vi "Measurement.TestLauncher.vi"() -> ()   [LabVIEW 2017]
doc: "JKI State Machine Objects (SMO) 1.0.0.5\nJKI - JKI\nCopyright (c) 2016, JKI"
uses:
  Measurement.Free.UI.lvclass
  D:/Program Files (x86)/National Instruments/LabVIEW 2017/vi.lib/JKI/JKI SMO/SMO/SMO.lvclass
  D:/Program Files (x86)/National Instruments/LabVIEW 2017/vi.lib/JKI/JKI SMO/SMO.UI/SMO.UI.lvclass
  Measurement.Free/Measurement.Free.lvclass
  Measurement.Free/Typedefs/Configuration--Cluster.ctl
  <vilib>/JKI/JKI SMO/SMO/SMO.lvclass
  <vilib>/JKI/JKI SMO/SMO.UI/SMO.UI.lvclass
panel:
  in  "Stop":bool
  # "SMO UI Test Launcher"
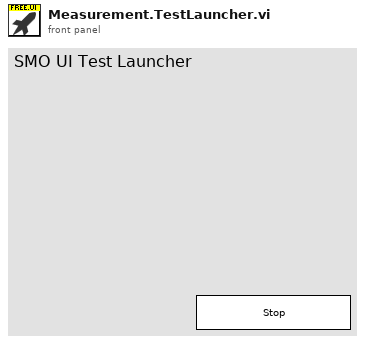
[diagram p1: front panel]
types:
  T1 = typedef "Measurement.Free.lvclass/Configuration--Cluster.ctl" = cluster{"Suffix":string}
  T2 = cluster{"SMO out":refnum<class "Measurement.Free.lvclass">}
  T3 = typedef "SMO.lvclass/Public Events.ctl" = cluster{"Error":refnum<user-event>, "State":refnum<user-event>, "Reserve State":refnum<user-event>}
  T4 = cluster{"Measurement.Free Public Events":refnum<event-registration>, "SMO.UI Public Events":refnum<event-registration>, "Event Registration Refnum":refnum<event-registration>}
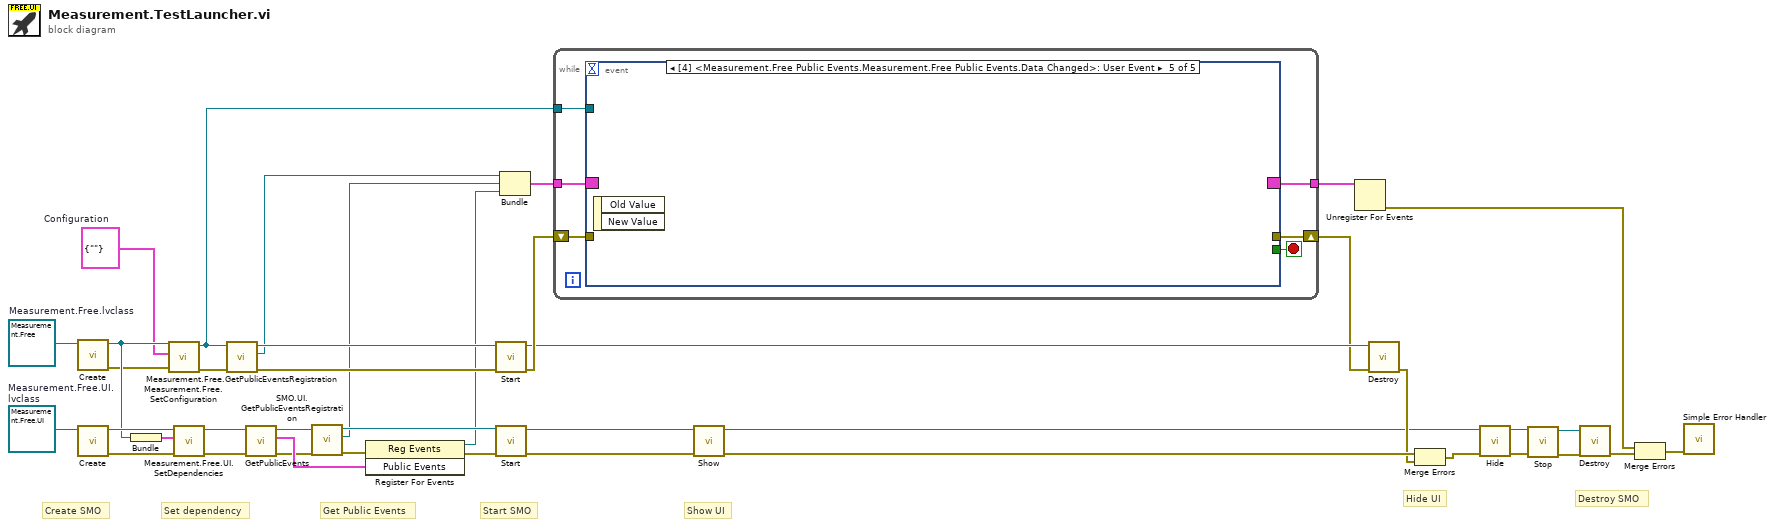
[diagram p0: block diagram]
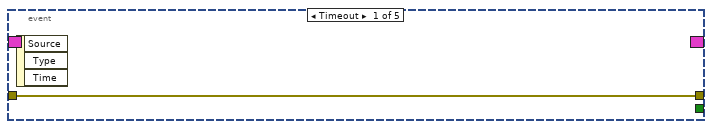
[diagram p2: hidden frame]
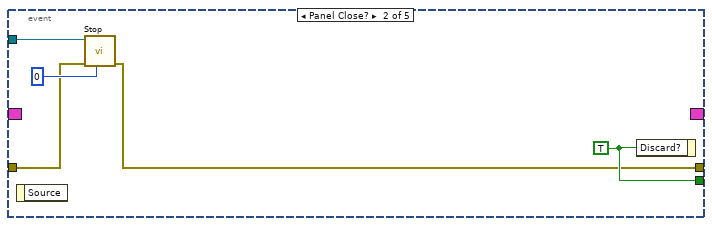
[diagram p3: hidden frame]
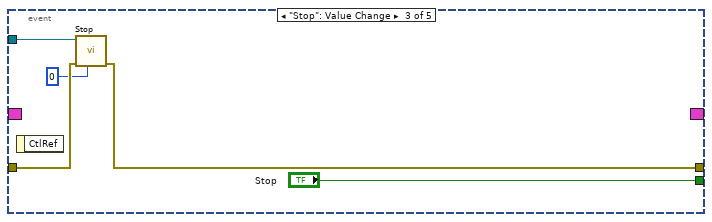
[diagram p4: hidden frame]
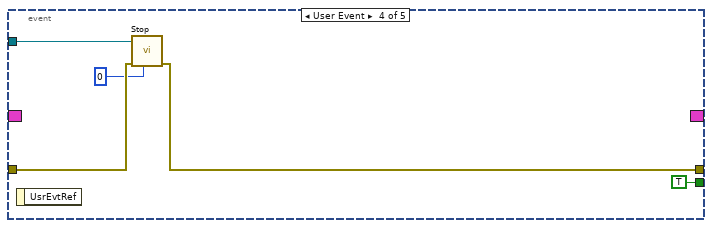
[diagram p5: hidden frame]
diagram:
  w25 = T1 {"Suffix"=""}  # Configuration
  w33 = refnum<class "Measurement.Free.lvclass"> refnum  # Measurement.Free.lvclass
  w34 = refnum<class "Measurement.Free.UI.lvclass"> refnum  # Measurement.Free.UI.lvclass
  # "Set dependency"
  # "Hide UI"
  # "Show UI"
  # "Get Public Events"
  # "Start SMO"
  # "Destroy SMO"
  # "Create SMO"
  n1 = call <vilib>:"Create.vi"("SMO"=w33) -> ("error out"=w26:errorcluster, "SMO out"=w27:refnum<class "Measurement.Free.lvclass">)  [unwired: 8 in, 1 out]
  n2 = call <vilib>:"Create.vi"("SMO"=w34) -> ("error out"=w30:errorcluster, "SMO out"=w32:refnum<class "Measurement.Free.UI.lvclass">)  [unwired: 8 in, 1 out]
  n3 = Bundle("SMO out"=w27) -> (w31:T2)  [unwired: 1 in]
  n4 = call "Measurement.Free.SetConfiguration.vi"("error in (no error)"=w26, "Configuration"=w25, "Measurement.Free"=w27) -> ("error out"=w10:errorcluster, "Measurement.Free out"=w11:refnum<class "Measurement.Free.lvclass">)  [unwired: 7 in]
  n5 = call "Measurement.Free.UI.SetDependencies.vi"("error in (no error)"=w30, "Dependencies"=w31, "Measurement.Free.UI in"=w32) -> ("error out"=w28:errorcluster, "Measurement.Free.UI out"=w29:refnum<class "Measurement.Free.UI.lvclass">)  [unwired: 7 in]
  n6 = call "Measurement.Free.GetPublicEventsRegistration.vi"("error in (no error)"=w10, "Measurement.Free"=w11) -> ("error out"=w8:errorcluster, "Measurement.Free Public Events"=w7:refnum<event-registration>, "Measurement.Free out"=w9:refnum<class "Measurement.Free.lvclass">)  [unwired: 7 in]
  n7 = call <vilib>:"GetPublicEvents.vi"("error in (no error)"=w28, "SMO"=w29) -> ("error out"=w5:errorcluster, "Public Events"=w35:T3, "SMO out"=w6:refnum<class "Measurement.Free.UI.lvclass">)  [unwired: 7 in]
  n8 = call <vilib>:"SMO.UI.GetPublicEventsRegistration.vi"("error in (no error)"=w5, "SMO.UI"=w6) -> ("error out"=w3:errorcluster, "SMO.UI Public Events"=w1:refnum<event-registration>, "SMO.UI out"=w4:refnum<class "Measurement.Free.UI.lvclass">)  [unwired: 7 in]
  n9 = register-events(error in=w3, w35) -> (reference out=w2:refnum<event-registration>, error out=w36:errorcluster)  [unwired: 1 in]
  n10 = call <vilib>:"Start.vi"("error in (no error)"=w8, "SMO"=w9) -> ("error out"=w22:errorcluster, "SMO out"=w21:refnum<class "Measurement.Free.lvclass">)  [unwired: 8 in]
  n11 = call <vilib>:"Start.vi"("error in (no error)"=w36, "SMO"=w4) -> ("error out"=w38:errorcluster, "SMO out"=w39:refnum<class "Measurement.Free.UI.lvclass">)  [unwired: 8 in]
  n12 = Bundle("Measurement.Free Public Events"=w7, "SMO.UI Public Events"=w1, "Event Registration Refnum"=w2) -> (w24:T4)  [unwired: 1 in]
  n13 = while {
    shift-right: [w46] -> w20
    shift-left: w22 -> [w45]
    tunnel: w24 -> [w42]
    tunnel: [w44] -> w23
    tunnel: w11 -> [w43]
    stop <- w47 stop-if-true
    n14 = event shown="[4] <Measurement.Free Public Events.Measurement.Free Public Events.Data Changed>: User Event" {
      selector: w42 -> [_ _ _ _ _]
      dyn-events: [_ _ _ _ _] -> w44
      timeout: _ -> [_ _ _ _ _]
      tunnel: [_ w53 "Stop" TRUE ("OK") _] -> w47
      tunnel: w43 -> [_ w52 w57 w63 _]
      tunnel: [w48 w49 w55 w61 _] -> w46
      tunnel: w45 -> [w48 w50 w56 w62 _]
      event Timeout {
        n15 = event-data() -> ()  [unwired: 1 in, 3 out]
      }
      event Panel Close? {
        w53 = TRUE ("OK")
        n16 = event-data() -> ()  [unwired: 1 in, 1 out]
        n17 = call <vilib>:"Stop.vi"("timeout in ms (-1)"=0, "error in (no error)"=w50, "SMO"=w52) -> ("error out"=w49:errorcluster)  [unwired: 7 in, 1 out]
        n18 = event-data("Discard?"=w53) -> ()  [unwired: 1 in, 1 out]
      }
      event "Stop": Value Change {
        n19 = event-data() -> ()  [unwired: 1 in, 1 out]
        n20 = call <vilib>:"Stop.vi"("timeout in ms (-1)"=0, "error in (no error)"=w56, "SMO"=w57) -> ("error out"=w55:errorcluster)  [unwired: 7 in, 1 out]
      }
      event User Event {
        n21 = event-data() -> ()  [unwired: 1 in, 1 out]
        n22 = call <vilib>:"Stop.vi"("timeout in ms (-1)"=0, "error in (no error)"=w62, "SMO"=w63) -> ("error out"=w61:errorcluster)  [unwired: 7 in, 1 out]
      }
      event User Event {
        n23 = event-data() -> ()  [unwired: 1 in, 2 out]
      }
    }
  }
  n24 = call <vilib>:"Show.vi"("error in (no error)"=w38, "SMO.UI"=w39) -> ("error out"=w37:errorcluster, "SMO.UI out"=w18:refnum<class "Measurement.Free.UI.lvclass">)  [unwired: 8 in]
  n25 = Unregister For Events(event registration refnum=w23) -> (error out=w41:errorcluster)  [unwired: 1 in]
  n26 = call <vilib>:"Destroy.vi"("error in (no error)"=w20, "SMO"=w21) -> ("error out"=w19:errorcluster)  [unwired: 9 in]
  n27 = Merge Errors(w37, w19) -> (w17:errorcluster)
  n28 = call <vilib>:"Hide.vi"("error in (no error)"=w17, "SMO.UI"=w18) -> ("error out"=w15:errorcluster, "SMO.UI out"=w16:refnum<class "Measurement.Free.UI.lvclass">)  [unwired: 8 in]
  n29 = call <vilib>:"Stop.vi"("error in (no error)"=w15, "SMO"=w16) -> ("error out"=w14:errorcluster, "SMO out"=w13:refnum<class "Measurement.Free.UI.lvclass">)  [unwired: 8 in]
  n30 = call <vilib>:"Destroy.vi"("error in (no error)"=w14, "SMO"=w13) -> ("error out"=w40:errorcluster)  [unwired: 9 in]
  n31 = Merge Errors(w41, w40) -> (w12:errorcluster)
  n32 = call <vilib>:"Simple Error Handler.vi"("error in (no error)"=w12) -> ()  [unwired: 4 in, 5 out]
